vi "ParseSWI.vi"(8 "error in (no error)":errorcluster, 9 "Master Device in":refnum<class "Master Device.lvclass">, 10 "Current Variables":T1[](array[typedef]), 11 "ArduinoDAC in":refnum<class "ArduinoDAC.lvclass">) -> (0 "error out":errorcluster, 2 "Master Device out":refnum<class "Master Device.lvclass">, 3 "ArduinoDAC out":refnum<class "ArduinoDAC.lvclass">)   [LabVIEW 2013, in "ArduinoDAC.lvclass"]
doc: "All specific devices will override ParseSWI method (i.e. you can delete the parent call)\n (1) Get devices data from private data\n (2) Get Slave Info (Ramp List) from Master Device\n (3) Parse data into \"prepared HWI\" which is in reverse order to match Ramp List."
uses:
  ArduinoDAC.lvclass
  TypeDefs/Active procedure variables.ctl
  Master Device/Master Device.lvclass
  ArduinoDAC.lvclass/ArduinoDAC.ctl
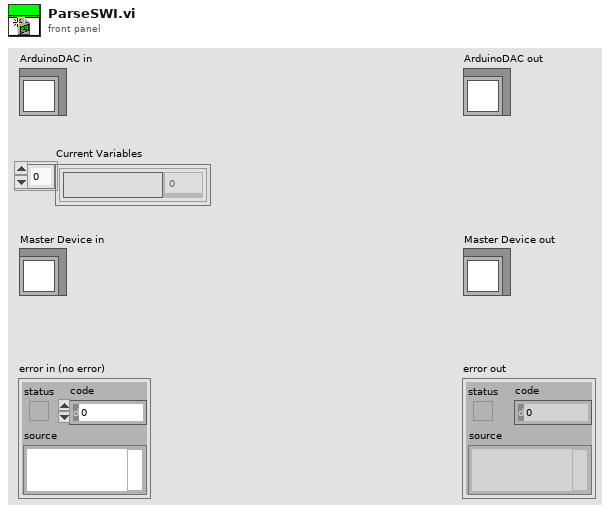
[diagram p1: front panel]
types:
  T1 = typedef "Active procedure variables.ctl" = cluster{"Procedure variable":string, "Value":dbl}
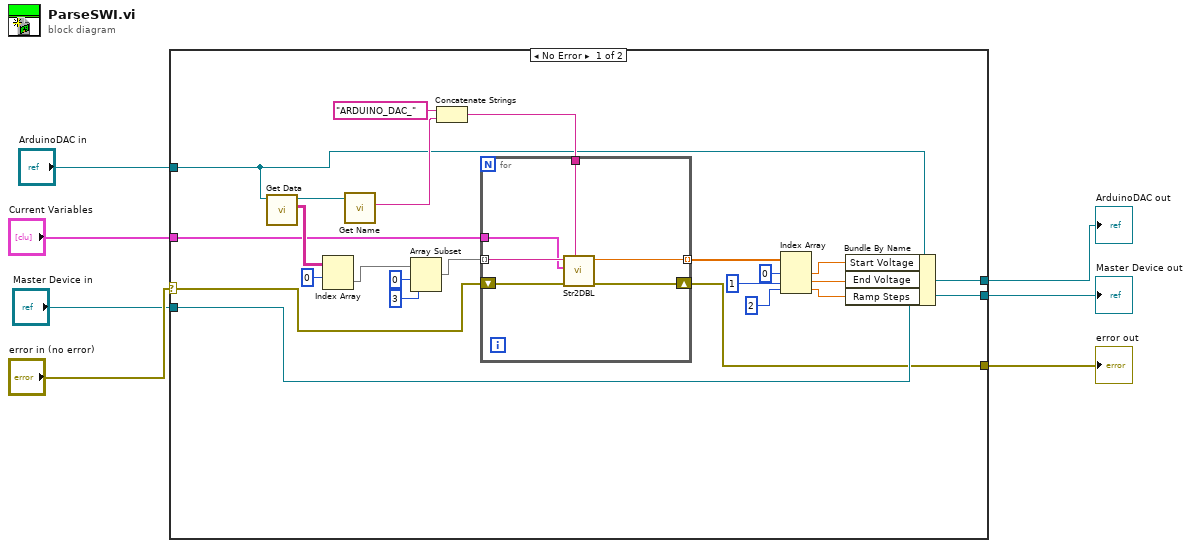
[diagram p0: block diagram]
diagram:
  n1 = case shown="No Error" "error in (no error)" {
    selector: "error in (no error)" -> [w9 w37]
    tunnel: "ArduinoDAC in" -> [w10 w39]
    tunnel: "Current Variables" -> [w23 _]
    tunnel: [w15 w39] -> w4
    tunnel: "Master Device in" -> [w14 w38]
    tunnel: [w14 w38] -> w2
    tunnel: [w8 w37] -> w1
    frame No Error {
      n2 = call-dynamic "Get Data.vi"("Device in"=w10) -> ("Table Indicator"=w29:string[][], "Device out"=w30:refnum<class "ArduinoDAC.lvclass">)  [unwired: 7 in, 1 out]
      n3 = Index Array(array=w29, index (row)=0) -> (element=w27:string[])  [unwired: 1 in]
      n4 = call-dynamic "Get Name.vi"("Device in"=w30) -> ("Name"=w21:string)  [unwired: 8 in, 2 out]
      n5 = Array Subset(array=w27, index=0, length=3 ("index")) -> (w24:string[])
      n6 = Concatenate Strings("ARDUINO_DAC_" ("string"), w21) -> (w20:string)
      n7 = for {
        tunnel: w24 -> [w36] mode=indexing
        tunnel: w23 -> [w35]
        tunnel: w20 -> [w34]
        tunnel: [w33] -> w19 mode=indexing
        shift-right: [w31] -> w8
        shift-left: w9 -> [w32]
        n8 = call "Str2DBL.vi"("Error Locator"=w34, "error in (no error)"=w32, "Current Variable settings"=w35, "formula"=w36) -> ("error out"=w31:errorcluster, "y value"=w33:dbl)  [unwired: 4 in]
      }
      n9 = Index Array(array=w19, index #1=0 ("index"), index #2=1 ("index"), index #3=2 ("index")) -> (element #1=w13:dbl, element #2=w12:dbl, element #3=w11:dbl)
      n10 = Bundle By Name(cluster=w10, "Start Voltage"=w13, "End Voltage"=w12, "Ramp Steps"=w11) -> (w15:refnum<class "ArduinoDAC.lvclass">)
    }
    frame Error {
    }
  }
  "error out" <- w1
  "ArduinoDAC out" <- w4
  "Master Device out" <- w2
